vi "HPF_First_Order_Sim.vi"(1 "x":dbl, 2 "fc(Hz)":dbl=0.20000000000000007 min=0.01 max=10.0 step=0.05 format="%_3f") -> (0 "y":dbl)   [LabVIEW 2012]
uses:
  <vilib>/Simulation/Implementation/Shared/SIMSCR Execution Mode.ctl
  <vilib>/Simulation/Scripting/Companion Diagram/SimConfigNode/SimParams.ctl
  <vilib>/Simulation/Scripting/Companion Diagram/SimConfigNode/_simSolvers.ctl
  <vilib>/Simulation/Param Hierarchy/Typedefs/SIMPH Param Control Actions.ctl
  <vilib>/Simulation/Implementation/Shared/NILVSim_ParamChanged.vi
  <vilib>/Simulation/ContinuousLinear/Implementation/NILVSim Transfer Function Direct.llb/SIM Transfer Function Direct (SISO).vi
  <vilib>/Simulation/Implementation/Shared/NILVSim_Manager.vi
  <vilib>/Simulation/Implementation/Shared/NILVSim_FinalizeModel.vi
  <vilib>/Simulation/Implementation/Shared/SIM Unbundle Sim Info.vi
  <vilib>/Utility/error.llb/Clear Errors.vi
  <vilib>/Simulation/Implementation/Shared/NILVSim_GetModelError.vi
  <vilib>/Simulation/Implementation/Shared/SIM SimErrorHandler.vi
  <vilib>/Simulation/Implementation/Shared/SIM Bundle Sim Info.vi
  <vilib>/Simulation/Implementation/Shared/NILVSim_Initialize.vi
  <vilib>/Simulation/Utility/Implementation/NILVSim Get Time and IsAcceptedStep.vi
  <vilib>/Simulation/Implementation/Shared/SIMSH Read Queue.vi
  <vilib>/Simulation/Scripting/Companion Diagram/SimConfigNode/SimDog.xnode
  <vilib>/Simulation/Implementation/XNodeFramework/SimXNode/SimX.xnode
  <vilib>/Simulation/Implementation/Shared/NI_SIM_Implementation.lvlib
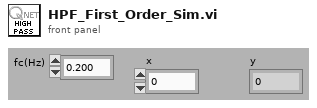
[diagram p1: front panel]
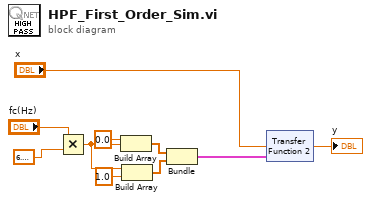
[diagram p0: block diagram]
diagram:
  n1 = Multiply(x="fc(Hz)", y=6.283185307179586 ("Constant")) -> (x*y=w6:dbl)
  n2 = Build Array(0.0 ("element 2"), w6) -> (w4:dbl[])
  n3 = Build Array ("Build Array 2")(w6, 1.0 ("element")) -> (w3:dbl[])
  n4 = Bundle(w4, w3) -> (w10:cluster{dbl[], dbl[]})  [unwired: 1 out]
  n5 = xnode ("Transfer Function 2")("input u(k)"="x", "Transfer Function"=w10) -> ("output y(k)"=→"y":dbl)  [unwired: 3 in, 1 out]
